vi "Write Model Number.vi"(8 "error in (no error)":errorcluster, 10 "Model Number":string, 11 "UUT in":refnum<class "UUT.lvclass">) -> (0 "error out":errorcluster, 3 "UUT out":refnum<class "UUT.lvclass">)   [LabVIEW 2021, in "Sequence Engine.lvlib" / "UUT.lvclass"]
uses:
  UUT.lvclass
  UUT.lvclass/UUT.ctl
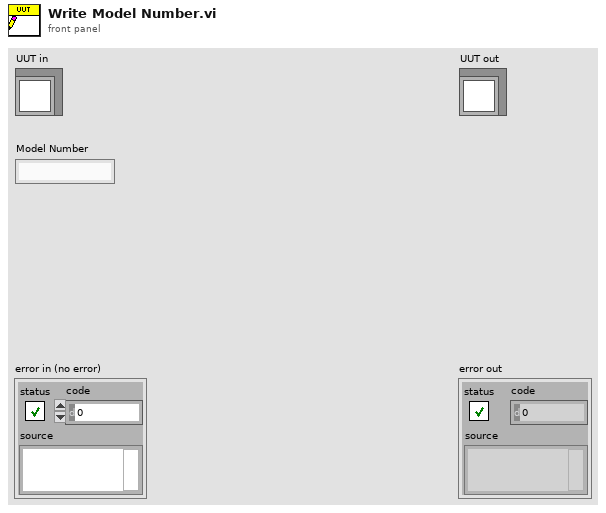
[diagram p1: front panel]
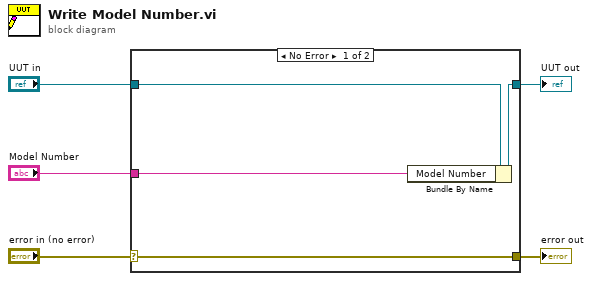
[diagram p0: block diagram]
diagram:
  n1 = case shown="No Error" "error in (no error)" {
    selector: "error in (no error)" -> [w9 w10]
    tunnel: [w9 w10] -> w4
    tunnel: [w7 w11] -> w2
    tunnel: "UUT in" -> [w8 w11]
    tunnel: "Model Number" -> [w6 _]
    frame No Error {
      n2 = Bundle By Name(cluster=w8, "Model Number"=w6) -> (w7:refnum<class "UUT.lvclass">)
    }
    frame Error {
    }
  }
  "error out" <- w4
  "UUT out" <- w2
